vi "Format Request Parameters.vi"(7 "Mode":T1, 11 "Request parameters":T2[](array[typedef])) -> (3 "Parameter string":string)   [LabVIEW 2015, in "NI_Azure_Core.lvlib"]
uses:
  NI_Azure_Core.lvlib
  Name Value Pair.ctl
  Format Request Parameters Mode.ctl
  <vilib>/Utility/error.llb/whitespace.ctl
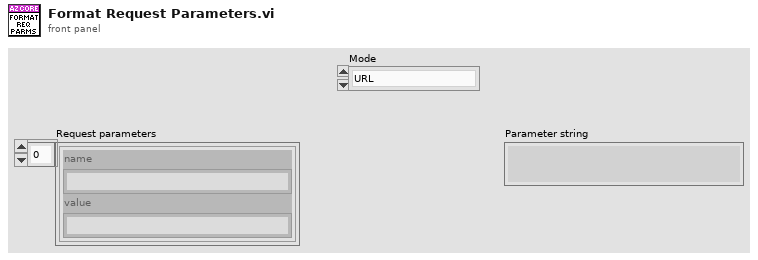
[diagram p1: front panel]
types:
  T1 = typedef "NI_Azure_Core.lvlib/Format Request Parameters Mode.ctl" = enum16{"URL", "Signing"}
  T2 = typedef "NI_Azure_Core.lvlib/Name Value Pair.ctl" = cluster{"name":string, "value":string}
  T3 = typedef "whitespace.ctl" = u16
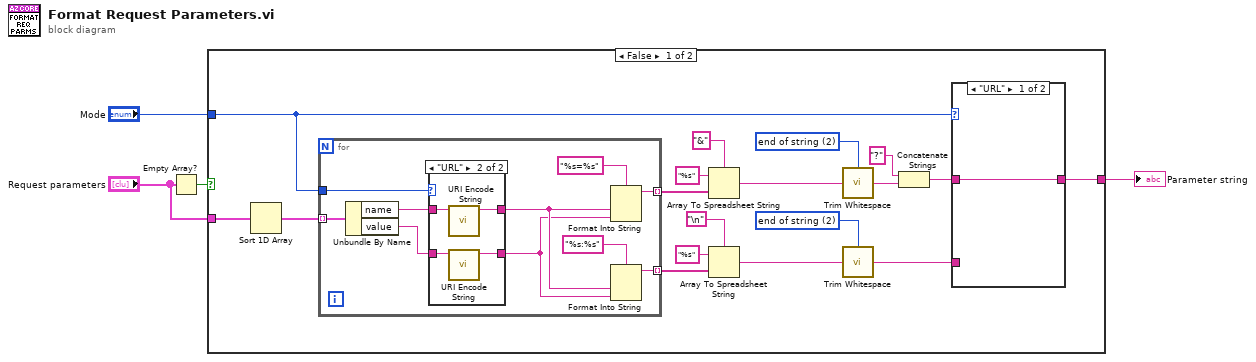
[diagram p0: block diagram]
diagram:
  n1 = Empty Array?(array="Request parameters") -> (empty?=w4:bool)
  n2 = case shown="False" w4 {
    tunnel: "Request parameters" -> [w22 _]
    tunnel: [w6 _] -> w2
    tunnel: "Mode" -> [w5 _]
    frame False {
      w13 = T3 2 items=["both", "start of string", "end of string"] ("location (both)")
      w14 = T3 2 items=["both", "start of string", "end of string"] ("location (both)")
      n3 = Sort 1D Array(array=w22) -> (sorted array=w9:T2[])
      n4 = for {
        tunnel: w9 -> [w34] mode=indexing
        tunnel: [w32] -> w21 mode=indexing
        tunnel: [w28] -> w16 mode=indexing
        tunnel: w5 -> [w25]
        n5 = Unbundle By Name(w34) -> ("name"=w30:string, "value"=w29:string)
        n6 = case shown="\"URL\"" w25 {
          tunnel: w30 -> [w36 w40]
          tunnel: w29 -> [w35 w39]
          tunnel: [w36 w38] -> w27
          tunnel: [w35 w37] -> w26
          frame Default {
          }
          frame "URL" {
            n7 = call "URI Encode String.vi"("Un-encoded String"=w40) -> ("UriEncoded String"=w38:string)  [unwired: 10 in]
            n8 = call "URI Encode String.vi"("Un-encoded String"=w39) -> ("UriEncoded String"=w37:string)  [unwired: 10 in]
          }
        }
        n9 = Format Into String(format string="%s=%s", w27, w26) -> (resulting string=w32:string)  [unwired: 2 in, 1 out]
        n10 = Format Into String(format string="%s:%s", w27, w26) -> (resulting string=w28:string)  [unwired: 2 in, 1 out]
      }
      n11 = Array To Spreadsheet String(delimiter (Tab)="&", array=w21, 3:"%s" ("format string")) -> (spreadsheet string=w18:string)
      n12 = Array To Spreadsheet String(delimiter (Tab)="\n", array=w16, 3:"%s" ("format string")) -> (spreadsheet string=w12:string)
      n13 = call <vilib>:"Trim Whitespace.vi"("string"=w18, "location (both)"=w14) -> ("trimmed string"=w11:string)
      n14 = call <vilib>:"Trim Whitespace.vi"("string"=w12, "location (both)"=w13) -> ("trimmed string"=w7:string)
      n15 = Concatenate Strings("?" ("format string"), w11) -> (w8:string)
      n16 = case shown="\"URL\"" w5 {
        tunnel: w8 -> [w23 _]
        tunnel: w7 -> [_ w24]
        tunnel: [w23 w24] -> w6
        frame "URL" {
        }
        frame "Signing" {
        }
      }
    }
    frame True {
    }
  }
  "Parameter string" <- w2
